vi "LC Refresh Control Path.vi"(8 "error in (no error)":errorcluster caption="Error In") -> (0 "error out":errorcluster caption="Error Out")   [LabVIEW 2020]
uses:
  LC Mode.ctl
  LC Single Control Information.ctl
  LC Global Mode.ctl
  c02344c7-2fc8-4ac7-8aa7-0093cc50af9f.vi
  <vilib>/Array/Sort 2D Array - Pop Stack.vi
  <vilib>/Array/Sort 2D Array - Push Stack.vi
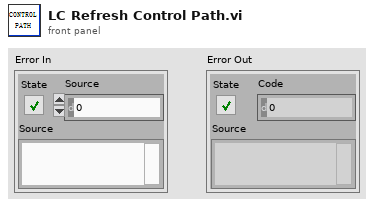
[diagram p1: front panel]
types:
  T1 = typedef "LC Single Control Information.ctl" = cluster{"VI Path":string, "VI Name":string, "Control Name":string, "Property Type":string, "Language":string, "Content":string}
  T2 = typedef "LC Global Mode.ctl" = enum16{"Init", "Read", "Write Language", "Write Version", "Save"}
  T3 = typedef "LC Mode.ctl" = enum16{"Init", "NONE", "Read", "Write", "Delete", "Clear", "Save"}
  T4 = typedef "LC Language Global.ctl" = cluster{"Language":string, "Version":string}
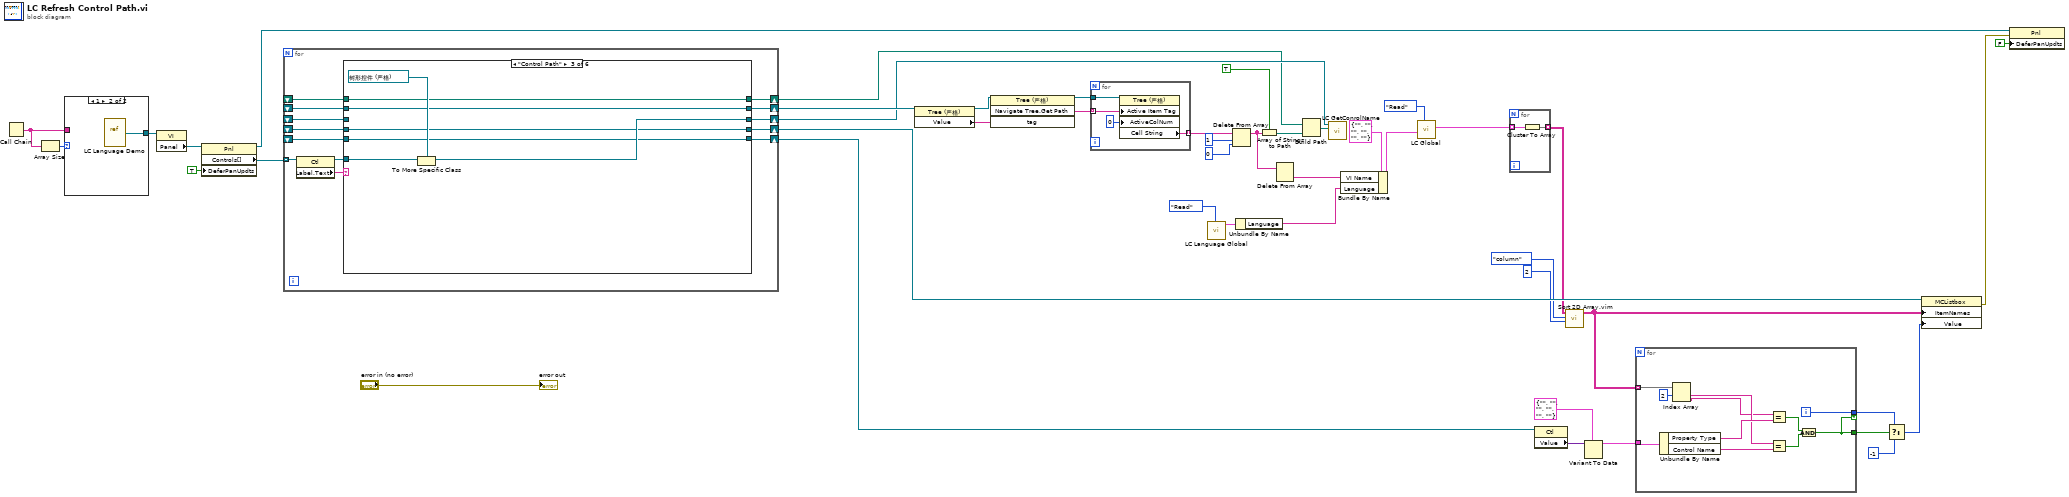
[diagram p0: block diagram]
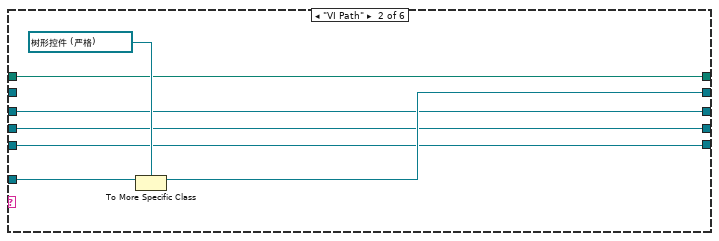
[diagram p3: hidden frame]
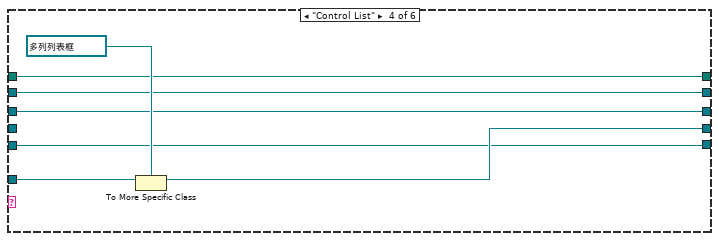
[diagram p4: hidden frame]
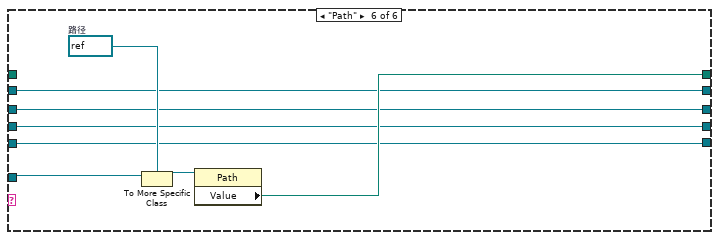
[diagram p6: hidden frame]
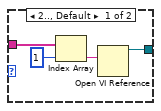
[diagram p7: hidden frame]
diagram:
  n1 = Call Chain() -> (call chain=w42:string[])
  n2 = Array Size(array=w42) -> (size(s)=w43:i32)
  n3 = case shown="1" w43 {
    tunnel: [w47 w50] -> w40
    tunnel: w42 -> [w46 _]
    frame 2.., Default {
      n4 = Index Array(array=w46, index=1 ("索引")) -> (element=w48:string)
      n5 = Open VI Reference(vi path=w48) -> (vi reference=w47:refnum<vi>)  [unwired: 5 in, 1 out]
    }
    frame 1 {
      n6 = vi-ref "LC Language Demo.vi"() -> (w50:refnum<vi>)
    }
  }
  n7 = property class="VI"(reference=w40) -> ("Panel"=w41:refnum<vi>)  [unwired: 1 in, 2 out]
  n8 = property class="Pnl"(reference=w41, "DeferPanUpdts"=TRUE ("延迟前面板更新")) -> (reference out=w1:refnum<vi>, "Controls[]"=w44:refnum<vi>[])  [unwired: 1 in, 1 out]
  n9 = for {
    tunnel: w44 -> [w63] mode=indexing
    shift-right: [w60] -> w28
    shift-left: _ -> [w59]
    shift-right: [w58] -> w30
    shift-left: _ -> [w57]
    shift-right: [w56] -> w29
    shift-left: _ -> [w55]
    shift-right: [w54] -> w17
    shift-left: _ -> [w53]
    shift-right: [w52] -> w15
    shift-left: _ -> [w51]
    n10 = property class="Ctl"(reference=w63) -> (reference out=w61:refnum<vi>, "Label.Text"=w62:string)  [unwired: 1 in, 1 out]
    n11 = case shown="\"Control Path\"" w62 {
      tunnel: w61 -> [_ w74 w81 w88 w90 w102]
      tunnel: [w68 w73 w80 w87 w94 w99] -> w60
      tunnel: w59 -> [w68 w73 w80 w87 w94 _]
      tunnel: [w67 w72 w79 w86 w93 w98] -> w58
      tunnel: w57 -> [w67 _ w79 w86 w93 w98]
      tunnel: [w66 w71 w78 w85 w92 w97] -> w56
      tunnel: w55 -> [w66 w71 _ w85 w92 w97]
      tunnel: [w65 w70 w77 w84 w91 w96] -> w54
      tunnel: w53 -> [w65 w70 w77 _ w91 w96]
      tunnel: [w64 w69 w76 w83 w90 w95] -> w52
      tunnel: w51 -> [w64 w69 w76 w83 _ w95]
      frame "eee", Default {
      }
      frame "VI Path" {
        n12 = To More Specific Class(target class=refnum<vi> refnum ("引用输出"), reference=w74) -> (specific class reference=w72:refnum<vi>)  [unwired: 1 in, 1 out]
      }
      frame "Control Path" {
        n13 = To More Specific Class(target class=refnum<vi> refnum ("引用输出"), reference=w81) -> (specific class reference=w78:refnum<vi>)  [unwired: 1 in, 1 out]
      }
      frame "Control List" {
        n14 = To More Specific Class(target class=refnum<vi> refnum ("引用输出"), reference=w88) -> (specific class reference=w84:refnum<vi>)  [unwired: 1 in, 1 out]
      }
      frame "Control_Info" {
      }
      frame "Path" {
        w101 = refnum<vi> refnum  # 路径
        n15 = To More Specific Class(target class=w101, reference=w102) -> (specific class reference=w100:refnum<vi>)  [unwired: 1 in, 1 out]
        n16 = property class="Path"(reference=w100) -> ("Value"=w99:path)  [unwired: 1 in, 2 out]
      }
    }
  }
  n17 = property class="Tree (严格)"(reference=w30) -> (reference out=w36:refnum<vi>, "Value"=w35:string)  [unwired: 1 in, 1 out]
  n18 = invoke class="Tree (严格)" method="Navigate Tree.Get Path"(reference=w36, "tag"=w35) -> (reference out=w39:refnum<vi>, "Navigate Tree:Get Path"=w37:string[])  [unwired: 2 in, 2 out]
  n19 = for {
    tunnel: w37 -> [w105] mode=indexing
    tunnel: [w104] -> w38 mode=indexing
    tunnel: w39 -> [w103]
    n20 = property class="Tree (严格)"(reference=w103, "Active Item Tag"=w105, "ActiveColNum"=0 ("活动单元格:活动列数")) -> ("Cell String"=w104:string)  [unwired: 1 in, 2 out]
  }
  n21 = call "LC Language Global.vi"("Mode"=LC_Global_Mode."Read") -> ("Read"=w20:T4)  [unwired: 9 in, 1 out]
  n22 = Delete From Array(array=w38, length=1 ("长度"), index=0 ("索引")) -> (array with subset deleted=w23:string[])  [unwired: 1 out]
  n23 = Unbundle By Name(w20) -> ("Language"=w19:string)
  n24 = Array of Strings to Path(0:w23, 1:TRUE ("相对")) -> (2:w34:path)
  n25 = Delete From Array(array=w23) -> (deleted portion=w22:string)  [unwired: 2 in, 1 out]
  n26 = Build Path(base path=w28, name or relative path=w34) -> (appended path=w33:path)
  n27 = call "LC GetConrolName.vi"("VI Path"=w33, "Treeref"=w29) -> ()  [unwired: 7 in, 3 out]
  n28 = Bundle By Name(cluster=T1 {"VI Path"="", "VI Name"="", "Control Name"="", "Property Type"="", "Language"="", "Content"=""} ("Write"), "VI Name"=w22, "Language"=w19) -> (w24:T1)
  n29 = call "LC Global.vi"("Mode"=LC_Mode."Read", "Write"=w24) -> ("Read"=w18:T1[])  [unwired: 7 in, 2 out]
  n30 = for {
    tunnel: w18 -> [w107] mode=indexing
    tunnel: [w108] -> w16 mode=indexing
    n31 = Cluster To Array(cluster=w107) -> (array=w108:string[])
  }
  n32 = property class="Ctl"(reference=w15) -> ("Value"=w13:variant)  [unwired: 1 in, 2 out]
  n33 = call "Sort 2D Array.vim"("index"=2, "dimension to index (column)"=enum16{"column", "row"}."column", "2D array"=w16) -> ("sorted 2D array"=w10:string[][])  [unwired: 7 in, 1 out]
  n34 = Variant To Data(type=T1 {"VI Path"="", "VI Name"="", "Control Name"="", "Property Type"="", "Language"="", "Content"=""} ("Control_Info"), Variant=w13) -> (data=w9:T1)  [unwired: 1 in, 1 out]
  n35 = for {
    tunnel: w10 -> [w112] mode=indexing
    tunnel: w9 -> [w119]
    tunnel: [w113] -> w8
    tunnel: [w114] -> w5 if=w113
    i -> [w114]
    n36 = Unbundle By Name(w119) -> ("Property Type"=w118:string, "Control Name"=w117:string)
    n37 = Index Array(array=w112, index #1=2 ("索引")) -> (element #1=w110:string, element #2=w109:string)  [unwired: 1 in]
    n38 = Equal?(x=w109, y=w118) -> (x = y?=w116:bool)
    n39 = Equal?(x=w110, y=w117) -> (x = y?=w115:bool)
    n40 = And(x=w116, y=w115) -> (x .and. y?=w113:bool)
  }
  n41 = Select(t=w5, s=w8, f=-1) -> (s? t:f=w7:i32)
  n42 = property class="MCListbox"(reference=w17, "ItemNames"=w10, "Value"=w7) -> (error out=w3:errorcluster)  [unwired: 1 in, 1 out]
  n43 = property class="Pnl"(reference=w1, error in=w3, "DeferPanUpdts"=FALSE ("延迟前面板更新")) -> ()  [unwired: 2 out]
  "error out" <- "error in (no error)"
